vi "File Name.vi"(8 "Error In":errorcluster, 9 "Trial Number":i32, 10 "Condition":string, 11 "Subject":string) -> (0 "Error Out":errorcluster, 3 "File Name":string)   [LabVIEW 2020, in "CollectionSupport.lvlib"]
uses:
  CollectionSupport.lvlib
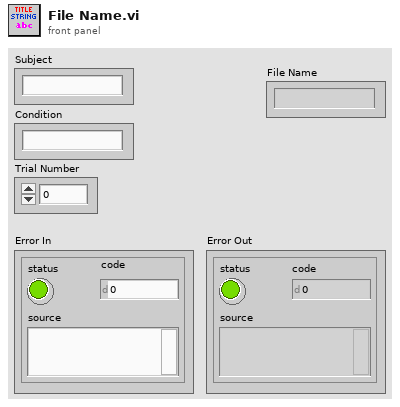
[diagram p1: front panel]
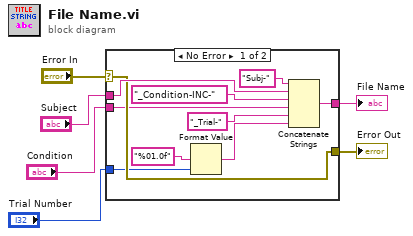
[diagram p0: block diagram]
diagram:
  n1 = case shown="No Error" "Error In" {
    selector: "Error In" -> [w13 w17]
    tunnel: [w13 w17] -> w5
    tunnel: "Trial Number" -> [w12 _]
    tunnel: "Subject" -> [w15 _]
    tunnel: "Condition" -> [w9 _]
    tunnel: [w14 _] -> w1
    frame No Error {
      n2 = Format Value(format string="%01.0f", value (0)=w12) -> (output string=w7:string)  [unwired: 1 in]
      n3 = Concatenate Strings("Subj-" ("string"), w15, "_Condition-INC-" ("string"), w9, "_Trial-" ("string"), w7) -> (w14:string)
    }
    frame Error {
    }
  }
  "Error Out" <- w5
  "File Name" <- w1
